vi "Write Board String.vi"(8 "error in (no error)":errorcluster, 10 "Board String":string, 11 "Map in":refnum<class "Map.lvclass">) -> (0 "error out":errorcluster, 3 "Map out":refnum<class "Map.lvclass">)   [LabVIEW 2019, in "Map.lvclass"]
uses:
  Map.lvclass
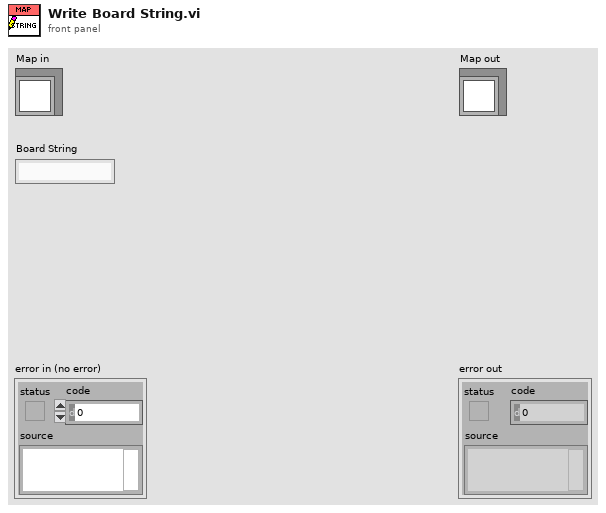
[diagram p1: front panel]
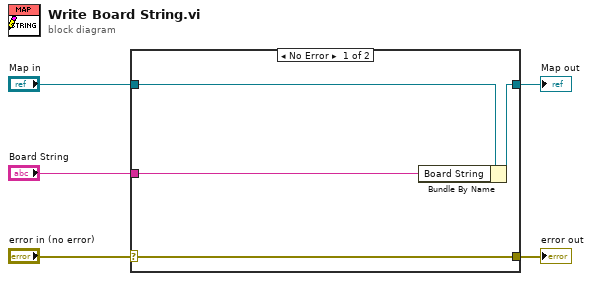
[diagram p0: block diagram]
diagram:
  n1 = case shown="No Error" "error in (no error)" {
    selector: "error in (no error)" -> [w9 w10]
    tunnel: [w9 w10] -> w4
    tunnel: [w7 w11] -> w2
    tunnel: "Map in" -> [w8 w11]
    tunnel: "Board String" -> [w6 _]
    frame No Error {
      n2 = Bundle By Name(cluster=w8, "Board String"=w6) -> (w7:refnum<class "Map.lvclass">)
    }
    frame Error {
    }
  }
  "error out" <- w4
  "Map out" <- w2
